vi "Rec_configure tdms.vi"(9 "文件名":string, 11 "数据存放路径":path) -> (3 "tdms out":refnum<k34>, 5 "文件路径":path)   [LabVIEW 2017]
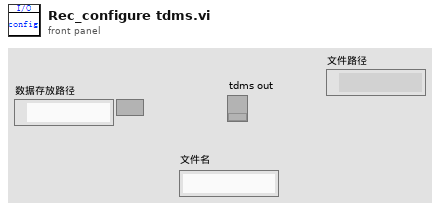
[diagram p1: front panel]
types:
  T1 = enum16{"open", "open or create", "create or replace", "create", "open (read-only)"}
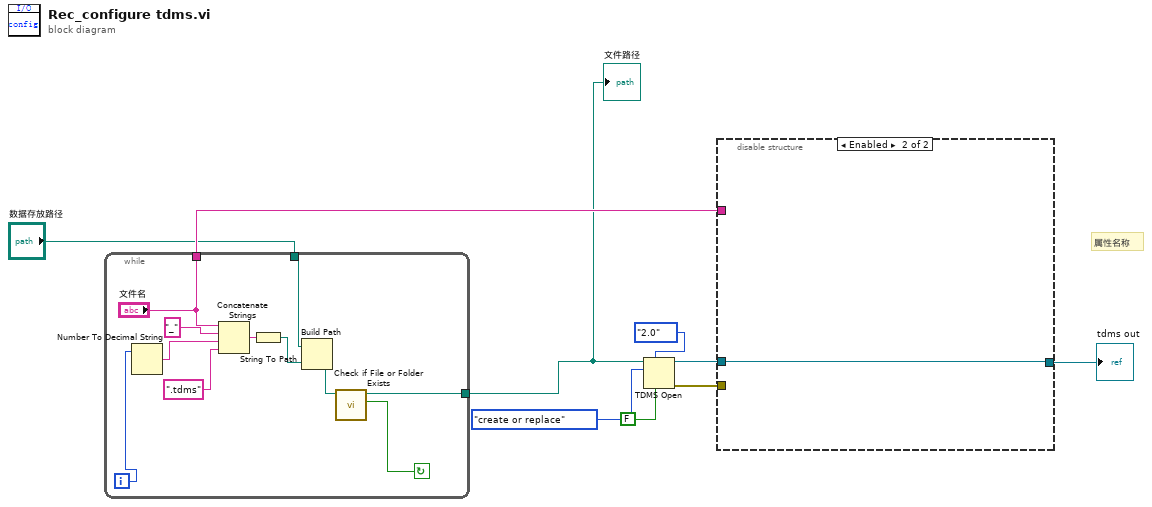
[diagram p0: block diagram]
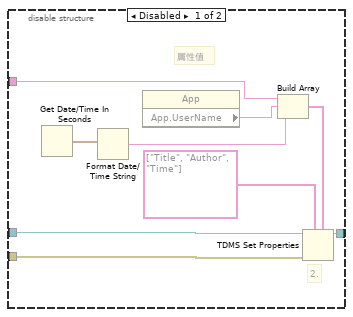
[diagram p2: hidden frame]
diagram:
  # "属性名称"
  n1 = while {
    tunnel: ["文件名"] -> w3
    tunnel: "数据存放路径" -> [w17]
    tunnel: [w12] -> w1
    i -> [w14]
    stop <- w16 continue-if-true
    n2 = Number To Decimal String(number=w14) -> (decimal integer string=w13:string)  [unwired: 1 in]
    n3 = Concatenate Strings("文件名", "_" ("string"), w13, ".tdms" ("字符串")) -> (w19:string)
    n4 = String To Path(string=w19) -> (path=w20:path)
    n5 = Build Path(base path=w17, name or relative path=w20) -> (appended path=w18:path)
    n6 = call <vilib>:"Check if File or Folder Exists.vi"("path"=w18) -> ("file or folder exists?"=w16:bool, "dup path"=w12:path)  [unwired: 8 in, 1 out]
  }
  "文件路径" <- w1
  n7 = TDMS Open(6:FALSE ("disable buffering (T)"), 7:enum16{"1.0", "2.0"}."2.0" ("file format version (2.0)"), 10:T1."create or replace" ("operation"), 11:w1) -> (0:w5:errorcluster, 3:w6:refnum<k34>)  [unwired: 3 in]
  n8 = disable-structure shown="Enabled" {
    disable-tunnel: w6 -> [w26 w30]
    disable-tunnel: w5 -> [w25 _]
    disable-tunnel: [w24 w30] -> w4
    disable-tunnel: w3 -> [w21 _]
    frame Disabled {
      # "属性值"
      # "2."
      n9 = Get Date/Time In Seconds() -> (seconds since 1Jan1904=w23:timestamp)
      n10 = Format Date/Time String(seconds (now)=w23) -> (date/time string=w22:string)  [unwired: 2 in]
      n11 = property class="App"() -> ("App.UserName"=w28:string)  [unwired: 2 in, 2 out]
      n12 = Build Array(w21, w28, w22) -> (w27:string[])
      n13 = TDMS Set Properties(5:w27, 7:string[] ["Title", "Author", "Time"] ("property names"), 8:w25, 11:w26) -> (3:w24:refnum<k34>)  [unwired: 5 out]
    }
    frame Enabled {
    }
  }
  "tdms out" <- w4
